vi "Get Loaded Plugins.vi"(8 "Error In":errorcluster, 11 "Factory Plugin Framework in":refnum<class "Factory Plugin Framework.lvclass">=refnum) -> (0 "Error Out":errorcluster, 2 "Loaded Plugins":T1(array[cluster]), 3 "Factory Plugin Framework out":refnum<class "Factory Plugin Framework.lvclass">)   [LabVIEW 2018, in "Factory Plugin Framework.lvlib" / "Factory Plugin Framework.lvclass"]
uses:
  Factory Plugin Framework.lvclass
  Factory Plugin Framework.lvclass/Factory Plugin Framework.ctl
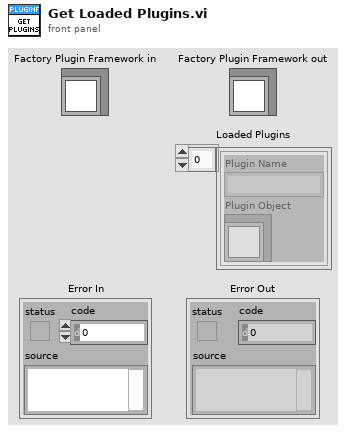
[diagram p1: front panel]
types:
  T1 = cluster{"Plugin Name":string, "Plugin Object":refnum<class>}[]
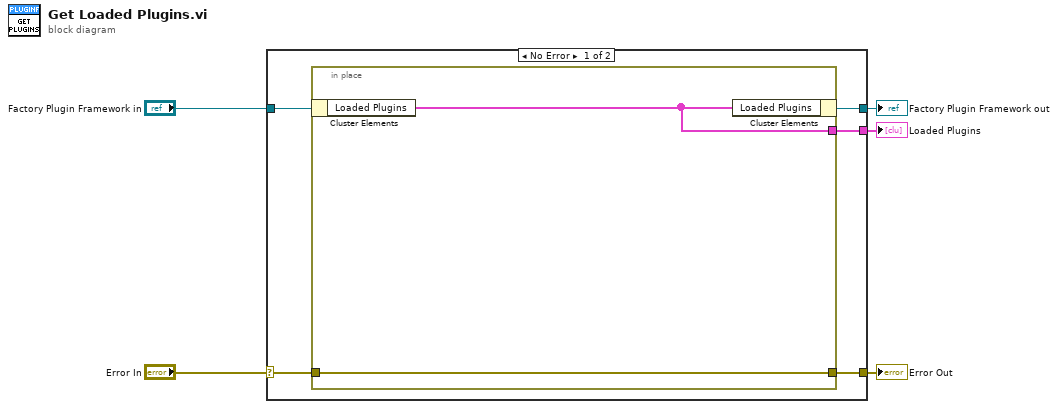
[diagram p0: block diagram]
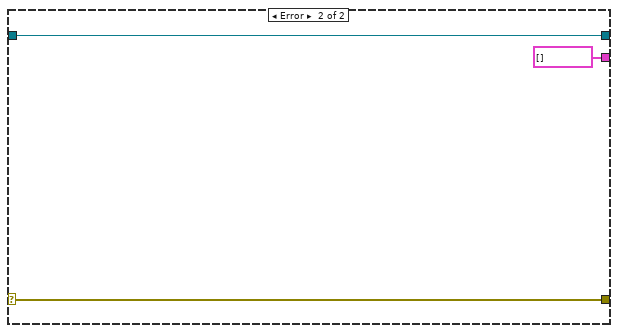
[diagram p2: hidden frame]
diagram:
  n1 = case shown="No Error" "Error In" {
    selector: "Error In" -> [w10 w15]
    tunnel: [w9 w15] -> w4
    tunnel: [w7 w14] -> w2
    tunnel: "Factory Plugin Framework in" -> [w8 w14]
    tunnel: [w6 T1 [] ("Private Methods:Loaded Plugins")] -> w1
    frame No Error {
      n2 = in-place {
        in-place-border: w10 -> [w12]
        in-place-border: [w12] -> w9
        in-place-border: [w11] -> w6
        n3 = in-place-cluster #1(w8) -> ("Loaded Plugins"=w11:T1)
        n4 = in-place-cluster #1("Loaded Plugins"=w11) -> (w7:refnum<class "Factory Plugin Framework.lvclass">)
      }
    }
    frame Error {
    }
  }
  "Error Out" <- w4
  "Factory Plugin Framework out" <- w2
  "Loaded Plugins" <- w1
